vi "mtect_regular_test.vi"() -> ()   [LabVIEW 2019]
uses:
  TEC LabVIEW Control Software v0.14/Source/LV Source/[meerstetter engineering TE Cooling]/TypeDefs/meTEC_ID 1200_Temperature is Stable.ctl
  TEC LabVIEW Control Software v0.14/Source/LV Source/[meerstetter engineering TE Cooling]/TypeDefs/meTEC_ID 104_Device Status.ctl
  TEC LabVIEW Control Software v0.14/Source/LV Source/[meerstetter engineering TE Cooling]/TypeDefs/meTEC_ID 2000_Input Selection.ctl
  TEC LabVIEW Control Software v0.14/Source/LV Source/[meerstetter engineering TE Cooling]/TypeDefs/meTEC_ID 50011_Object Target Temperature Source Selection.ctl
  TEC LabVIEW Control Software v0.14/Source/LV Source/[meerstetter engineering TE Cooling]/TypeDefs/meTEC_ID 50000_Live Enable.ctl
  MTec_class/MTec.lvclass
panel:
  out "error out":errorcluster
  in  "Config Data":T4={"meTEC_CH1_Input Selection (ID 2000)"=2, "meTEC_CH2_Input Selection (ID 2000)"=2, "meTEC_CH1_Object Target Temp. Source Selection (ID 50011)"=0, "meTEC_CH2_Object Target Temp. Source Selection (ID 50011)"=0, "meTEC_CH1_Live Enable (ID 50000)"=0, "meTEC_CH2_Live Enable (ID 50000)"=0, "meTEC_CH1_Object Target Temperature (ID 3000 / 50012) [°C]"=23.0, "meTEC_CH2_Object Target Temperature (ID 3000 / 50012) [°C]"=23.0, "meTEC_CH1_Live Set Current (ID 50001) [A]"=0.0, "meTEC_CH2_Live Set Current (ID 50001) [A]"=0.0, "meTEC_CH1_Live Set Voltage (ID 50002) [V]"=0.0, "meTEC_CH2_Live Set Voltage (ID 50002) [V]"=0.0} {"meTEC_CH2_Live Set Voltage (ID 50002) [V]" min=0.0 max=22.000001907348633 step=0.001 format="%#.3f"; "meTEC_CH1_Live Set Voltage (ID 50002) [V]" min=0.0 max=0.0 step=0.001 format="%#.3f"; "meTEC_CH2_Live Set Current (ID 50001) [A]" min=-10.0 max=10.0 step=0.001 format="%#.3f"; "meTEC_CH1_Live Set Current (ID 50001) [A]" min=0.0 max=0.0 step=0.001 format="%#.3f"; "meTEC_CH2_Object Target Temperature (ID 3000 / 50012) [°C]" min=-273.0 max=1000.0 step=0.001 format="%#.3f"; "meTEC_CH1_Object Target Temperature (ID 3000 / 50012) [°C]" min=0.0 max=0.0 step=0.001 format="%#.3f"; "meTEC_CH2_Live Enable (ID 50000)" items=["Disabled (Reset State)", "Enabled"]; "meTEC_CH1_Live Enable (ID 50000)" items=["Disabled (Reset State)", "Enabled"]; "meTEC_CH2_Object Target Temp. Source Selection (ID 50011)" items=["Parameter ID 3000 (Reset State)", "Parameter ID 50012"]; "meTEC_CH1_Object Target Temp. Source Selection (ID 50011)" items=["Parameter ID 3000 (Reset State)", "Parameter ID 50012"]; "meTEC_CH2_Input Selection (ID 2000)" items=["Static Current / Voltage", "Live Current / Voltage", "Temperature Controller"]; "meTEC_CH1_Input Selection (ID 2000)" items=["Static Current / Voltage", "Live Current / Voltage", "Temperature Controller"]}
  out "MtecData":T7={"meTEC_CH2_Temperature Stability"=1, "meTEC_CH2_Act. Output Current [A]"=0.0, "meTEC_CH2_Act. Output Voltage [V]"=0.0, "meTEC_CH2_Object Temperature [°C]"=0.0, "meTEC_CH2_Sink Temperature [°C]"=0.0, "meTEC_CH1_Error Parameter"=0, "meTEC_CH1_Error Instance"=0, "meTEC_CH1_Error No."=0, "meTEC_CH1_Device Status"=1, "meTEC_CH1_Temperature Stability"=1, "meTEC_CH1_Act. Output Current [A]"=0.0, "meTEC_CH1_Act. Output Voltage [V]"=0.0, "meTEC_CH1_Object Temperature [°C]"=0.0, "meTEC_CH1_Sink Temperature [°C]"=0.0} {"meTEC_CH1_Sink Temperature [°C]" format="%.3f"; "meTEC_CH1_Object Temperature [°C]" format="%.3f"; "meTEC_CH1_Act. Output Voltage [V]" format="%.3f"; "meTEC_CH1_Act. Output Current [A]" format="%.3f"; "meTEC_CH1_Temperature Stability" items=["Temperature regulation is not active", "Is not stable", "Is stable"]; "meTEC_CH1_Device Status" items=["Initializing", "Ready", "Run", "Error", "Bootloader", "Reset in Progress"]; "meTEC_CH2_Sink Temperature [°C]" format="%.3f"; "meTEC_CH2_Object Temperature [°C]" format="%.3f"; "meTEC_CH2_Act. Output Voltage [V]" format="%.3f"; "meTEC_CH2_Act. Output Current [A]" format="%.3f"; "meTEC_CH2_Temperature Stability" items=["Temperature regulation is not active", "Is not stable", "Is stable"]}
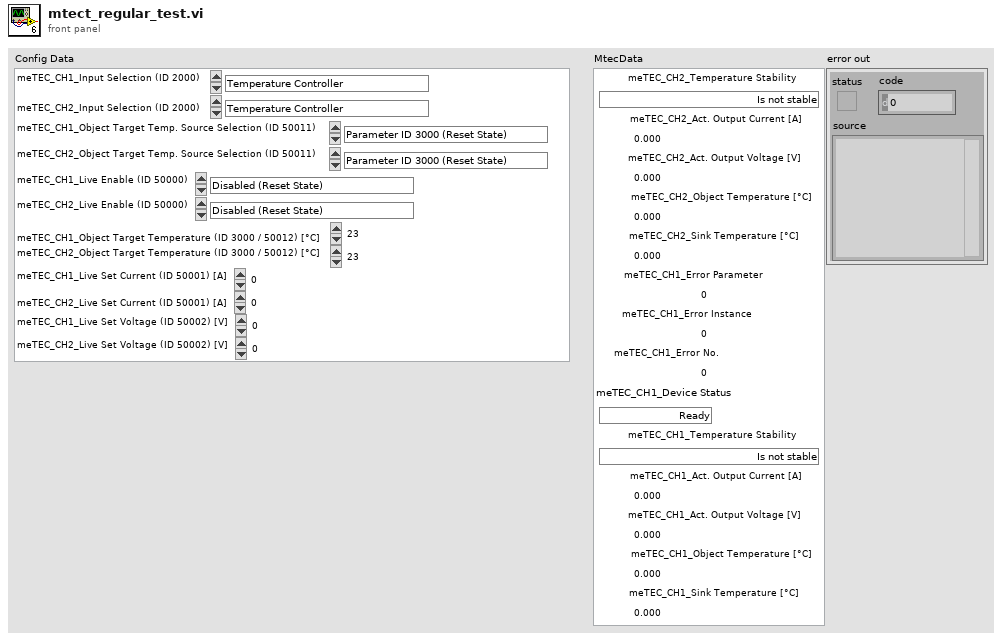
[diagram p1: front panel]
types:
  T1 = typedef "meTEC_ID 2000_Input Selection.ctl" = i32
  T2 = typedef "meTEC_ID 50011_Object Target Temperature Source Selection.ctl" = i32
  T3 = typedef "meTEC_ID 50000_Live Enable.ctl" = i32
  T4 = cluster{"meTEC_CH1_Input Selection (ID 2000)":T1, "meTEC_CH2_Input Selection (ID 2000)":T1, "meTEC_CH1_Object Target Temp. Source Selection (ID 50011)":T2, "meTEC_CH2_Object Target Temp. Source Selection (ID 50011)":T2, "meTEC_CH1_Live Enable (ID 50000)":T3, "meTEC_CH2_Live Enable (ID 50000)":T3, "meTEC_CH1_Object Target Temperature (ID 3000 / 50012) [°C]":dbl, "meTEC_CH2_Object Target Temperature (ID 3000 / 50012) [°C]":dbl, "meTEC_CH1_Live Set Current (ID 50001) [A]":dbl, "meTEC_CH2_Live Set Current (ID 50001) [A]":dbl, "meTEC_CH1_Live Set Voltage (ID 50002) [V]":dbl, "meTEC_CH2_Live Set Voltage (ID 50002) [V]":dbl}
  T5 = typedef "meTEC_ID 1200_Temperature is Stable.ctl" = i32
  T6 = typedef "meTEC_ID 104_Device Status.ctl" = i32
  T7 = cluster{"meTEC_CH2_Temperature Stability":T5, "meTEC_CH2_Act. Output Current [A]":dbl, "meTEC_CH2_Act. Output Voltage [V]":dbl, "meTEC_CH2_Object Temperature [°C]":dbl, "meTEC_CH2_Sink Temperature [°C]":dbl, "meTEC_CH1_Error Parameter":i32, "meTEC_CH1_Error Instance":i32, "meTEC_CH1_Error No.":i32, "meTEC_CH1_Device Status":T6, "meTEC_CH1_Temperature Stability":T5, "meTEC_CH1_Act. Output Current [A]":dbl, "meTEC_CH1_Act. Output Voltage [V]":dbl, "meTEC_CH1_Object Temperature [°C]":dbl, "meTEC_CH1_Sink Temperature [°C]":dbl}
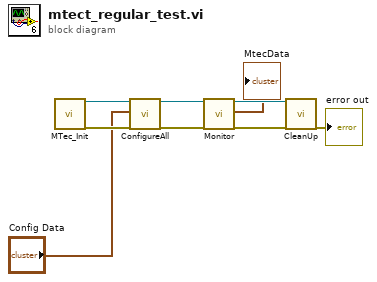
[diagram p0: block diagram]
diagram:
  n1 = call "MTec_Init.vi"() -> ("object out"=w9:refnum<class "MTec.lvclass">, "error out"=w6:errorcluster)  [unwired: 18 in]
  n2 = call-dynamic "ConfigureAll.vi"("object in"=w9, "Config Data"="Config Data", "error in (no error)"=w6) -> ("object out"=w8:refnum<class "MTec.lvclass">, "error out"=w5:errorcluster)  [unwired: 15 in]
  n3 = call-dynamic "Monitor.vi"("object in"=w8, "error in (no error)"=w5) -> ("object out"=w7:refnum<class "MTec.lvclass">, "MtecData"=→"MtecData":T7, "error out"=w4:errorcluster)  [unwired: 15 in]
  n4 = call-dynamic "CleanUp.vi"("object in"=w7, "error in (no error)"=w4) -> ("error out"=→"error out":errorcluster)  [unwired: 16 in, 1 out]
